vi "Write TCP Connection Info.vi"(8 "error in (no error)":errorcluster, 10 "TCP Connection Info":T1={"Server Address"="", "Port"=0, "Timeout (ms)"=60000, "Retry-interval (ms)"=5}, 11 "Function in":refnum<class "Function.lvclass">) -> (0 "error out":errorcluster, 3 "Function out":refnum<class "Function.lvclass">)   [LabVIEW 2016, in "Function Actor.lvlib" / "Function.lvclass"]
uses:
  <userlib>/Common Components/Function Actor/Function.lvclass
  <userlib>/Common Components/Function Actor/TCP connection info.ctl
  <userlib>/Common Components/Function Actor/Function.lvclass/Function.ctl
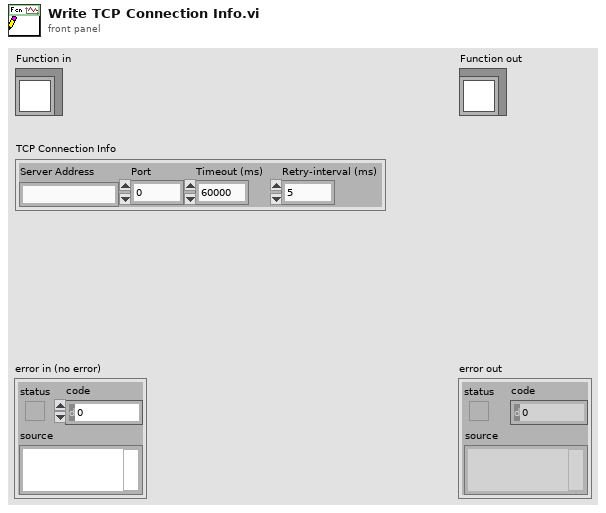
[diagram p1: front panel]
types:
  T1 = typedef "Function Actor.lvlib/Function.lvclass/TCP connection info.ctl" = cluster{"Server Address":string, "Port":u16, "Timeout (ms)":i32, "Retry-interval (ms)":i32}
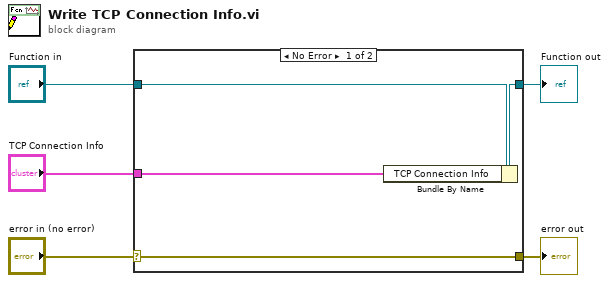
[diagram p0: block diagram]
diagram:
  n1 = case shown="No Error" "error in (no error)" {
    selector: "error in (no error)" -> [w9 w10]
    tunnel: [w9 w10] -> w4
    tunnel: [w7 w11] -> w2
    tunnel: "Function in" -> [w8 w11]
    tunnel: "TCP Connection Info" -> [w6 _]
    frame No Error {
      n2 = Bundle By Name(cluster=w8, "TCP Connection Info"=w6) -> (w7:refnum<class "Function.lvclass">)
    }
    frame Error {
    }
  }
  "error out" <- w4
  "Function out" <- w2
